vi "Point-Plane distance.vi"(3 "Plane normal (unit)":sgl[](array[numeric]), 4 "Point on plane":sgl[](array[numeric]), 5 "Point":sgl[](array[numeric])) -> (0 "Projected point on plane (along normal)":sgl[](array[numeric]), 1 "| Distance |":sgl, 2 "Distance vector (from plane)":sgl[](array[numeric]))   [LabVIEW 2014]
panel:
  # "PN 12/01/2015"
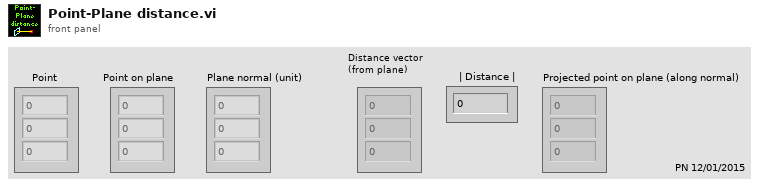
[diagram p1: front panel]
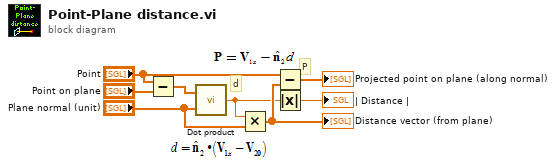
[diagram p0: block diagram]
diagram:
  # "P"
  # "d"
  n1 = Subtract(x="Point", y="Point on plane") -> (x-y=w8:sgl[])
  n2 = call "Dot product.vi"("B"="Plane normal (unit)", "A"=w8) -> ("A . B"=w2:sgl)
  n3 = Multiply(x=w2, y="Plane normal (unit)") -> (x*y=w3:sgl[])
  "Distance vector (from plane)" <- w3
  n4 = Subtract(x="Point", y=w3) -> (x-y=→"Projected point on plane (along normal)":sgl[])
  n5 = Absolute Value(x=w2) -> (abs(x)=→"| Distance |":sgl)
